vi "WS1021 Multi DUT Calculated Header.vi"(8 "Error In":errorcluster) -> (0 "Error Out":errorcluster, 3 "Name Calculated Header":string[](array[string]))   [LabVIEW 2017]
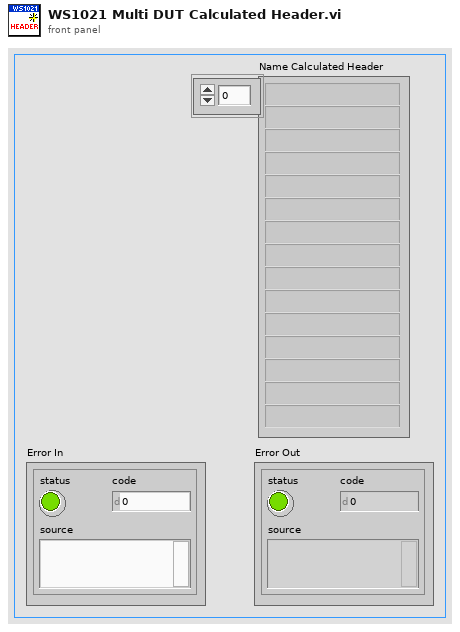
[diagram p1: front panel]
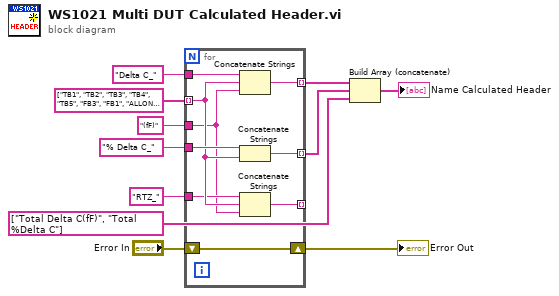
[diagram p0: block diagram]
diagram:
  n1 = for {
    tunnel: string[] ["TB1", "TB2", "TB3", "TB4", "TB5", "FB3", "FB1", "ALLON R3", "TB6", "TB7", "TB8", "TB9", "TB10", "TB11", "FB2", "ALLON R2"] -> [w16] mode=indexing
    tunnel: [w20] -> w4 mode=indexing
    tunnel: [w19] -> w3 mode=indexing
    tunnel: [w18] -> _ mode=indexing
    tunnel: "% Delta C_" ("string") -> [w17]
    tunnel: "RTZ_" ("string") -> [w15]
    tunnel: "Delta C_" ("string") -> [w14]
    tunnel: "(fF)" ("string") -> [w13]
    shift-right: [w12] -> w5
    shift-left: "Error In" -> [w12]
    n2 = Concatenate Strings(w14, w16, w13) -> (w20:string)
    n3 = Concatenate Strings(w17, w16) -> (w19:string)
    n4 = Concatenate Strings(w15, w16, w13) -> (w18:string)
  }
  "Error Out" <- w5
  n5 = Build Array (concatenate)(w4, w3, string[] ["Total Delta C(fF)", "Total %Delta C"]) -> (→"Name Calculated Header":string[])
